vi "setCounterMode.vi"(2 "error in (no error)":errorcluster, 3 "Mode":dbl, 4 "BK1823ACounter.lvclass":refnum<class "BK1823ACounter.lvclass">) -> (0 "error out":errorcluster, 1 "BK1823ACounter.lvclass 2":refnum<class "BK1823ACounter.lvclass">)   [LabVIEW 2009, in "Hardware.lvlib" / "frequencyCounters.lvlib" / "BK1823ACounter.lvclass"]
uses:
  BK1823ACounter.lvclass
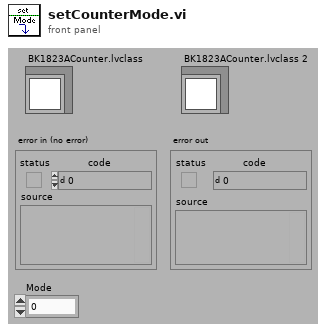
[diagram p1: front panel]
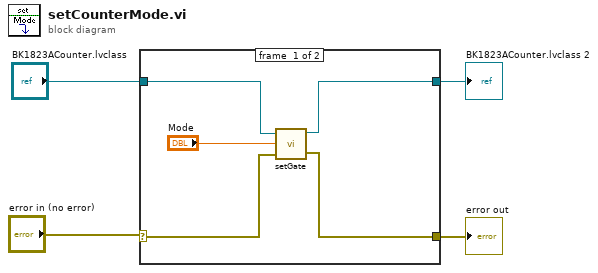
[diagram p0: block diagram]
diagram:
  n1 = case shown="No Error" "error in (no error)" {
    selector: "error in (no error)" -> [w6 w11]
    tunnel: [w5 w11] -> w3
    tunnel: "BK1823ACounter.lvclass" -> [w8 w10]
    tunnel: [w7 w10] -> w1
    frame #0 {
      n2 = call "setGate.vi"("error in (no error)"=w6, "Numeric"="Mode", "BK1823ACounter.lvclass"=w8) -> ("error out"=w5:errorcluster, "BK1823ACounter.lvclass 2"=w7:refnum<class "BK1823ACounter.lvclass">)
    }
    frame #1 {
    }
  }
  "error out" <- w3
  "BK1823ACounter.lvclass 2" <- w1
